vi "ReadTiffPage_text.vi"(0 "TIFF file":T2 {"BigTiff,Endian" items=["Big-Endian"=0, "Native"=1, "Little-Endian"=2, "BigTiff-Big-Endian"=256, "Bigtiff,Native"=257, "Biftiff,Littleendian"=258]}, 2 "IFDoffset":i64, 3 "error in":errorcluster) -> (6 "TIFF file out":T2 {"BigTiff,Endian" items=["Big-Endian"=0, "Native"=1, "Little-Endian"=2, "BigTiff-Big-Endian"=256, "Bigtiff,Native"=257, "Biftiff,Littleendian"=258]}, 8 "string":string, 9 "Next offset":i64, 10 "error out":errorcluster)   [LabVIEW 2011]
uses:
  IFD.ctl
  GetTagValues_U8s.vi
panel:
  out "Byte-Reihenfolge (0:Big-Endian, Netzwerkreihenfolge)":T1(ring)=enum."native, host order"
  out "Directory Entries":T3[](array[typedef])
  out "IFDs":u16
  # "seems to work!"
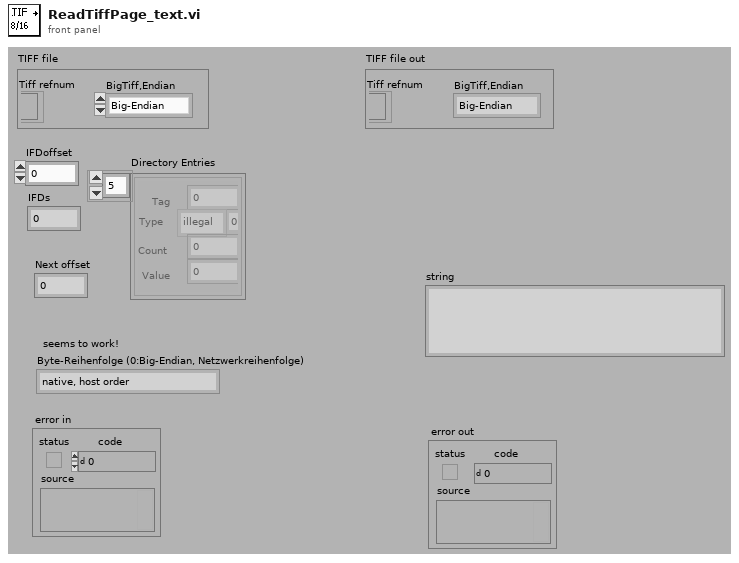
[diagram p1: front panel]
types:
  T1 = enum16{"big-endian, network order", "native, host order", "little-endian"}
  T2 = cluster{"Tiff refnum":refnum<file>, "BigTiff,Endian":u16}
  T3 = typedef "IFD.ctl" = cluster{"Tag":u16, "Type":enum16{"illegal", "Byte", "Ascii", "Short", "Long", "Rational", "SByte", "Undefined", "SShort", "SLong", "SRational 2xSLong", "Float 4byte", "Double 8Byte", "No13", "No14", "No15", "U64", "I64", "U64-IFD8"}, "Count":u64, "Value":u64}
  T4 = cluster{"Tag":u16, "Type":enum16{"illegal", "Byte", "Ascii", "Short", "Long", "Rational", "SByte", "Undefined", "SShort", "SLong", "SRational 2xSLong", "Float 4byte", "Double 8Byte"}, "Count":u32, "Value":u32}
  T5 = cluster{"Tag":u16, "Type":enum16{"illegal", "Byte", "Ascii", "Short", "Long", "Rational", "SByte", "Undefined", "SShort", "SLong", "SRational 2xSLong", "Float 4byte", "Double 8Byte"}, "Count":u32, "Value":u32}[]
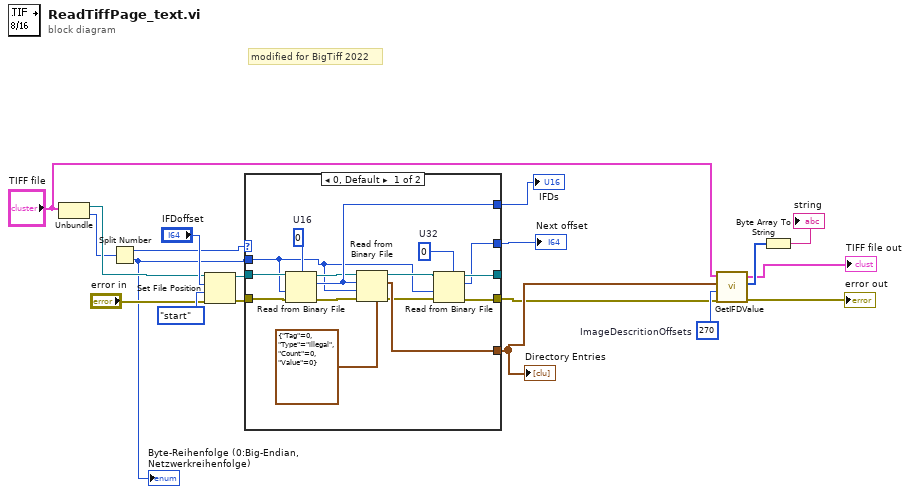
[diagram p0: block diagram]
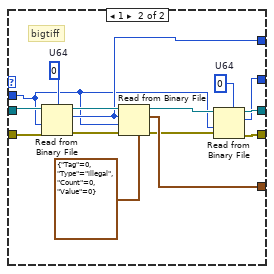
[diagram p2: hidden frame]
diagram:
  w14 = u16 270  # ImageDescritionOffsets
  # "modified for BigTiff 2022"
  n1 = Unbundle("TIFF file") -> ("Tiff refnum"=w16:refnum<file>, "BigTiff,Endian"=w12:u16)
  n2 = Split Number(x=w12) -> (hi(x)=w6:u8, lo(x)=w5:u8)
  "Byte-Reihenfolge (0:Big-Endian, Netzwerkreihenfolge)" <- w5
  n3 = Set File Position(offset (in bytes) (0)="IFDoffset", refnum=w16, from (0:start)=enum16{"start", "end", "current"}."start" ("pos mode (0:2)"), error in="error in") -> (refnum out=w7:refnum<file>, error out=w8:errorcluster)
  n4 = case shown="0, Default" w6 {
    tunnel: [w33 w43] -> w1
    tunnel: w8 -> [w32 w45]
    tunnel: w7 -> [w31 w44]
    tunnel: [w24 w38] -> _
    tunnel: [w23 w40] -> w3
    tunnel: [w28 w42] -> w4
    tunnel: w5 -> [w20 w37]
    tunnel: [w22 w35] -> w2
    frame 0, Default {
      w21 = u32 0  # U32
      w34 = u16 0  # U16
      n5 = Read from Binary File(5:w34, 8:w32, 9:w20, 11:w31) -> (0:w29:errorcluster, 2:w33:u16, 3:w30:refnum<file>)  [unwired: 3 out]
      n6 = Read from Binary File(5:T4 {"Tag"=0, "Type"=enum."illegal", "Count"=0, "Value"=0} ("Cluster"), 8:w29, 9:w20, 10:w33, 11:w30) -> (0:w26:errorcluster, 2:w28:T5, 3:w25:refnum<file>)  [unwired: 2 out]
      n7 = Read from Binary File(5:w21, 8:w26, 9:w20, 11:w25) -> (0:w23:errorcluster, 2:w22:u32, 3:w24:refnum<file>)  [unwired: 3 out]
    }
    frame 1 {
      w36 = u64 0  # U64
      w49 = u64 0  # U64
      # "bigtiff"
      n8 = Read from Binary File(5:w49, 8:w45, 9:w37, 11:w44) -> (0:w47:errorcluster, 2:w43:u64, 3:w48:refnum<file>)  [unwired: 3 out]
      n9 = Read from Binary File(5:T3 {"Tag"=0, "Type"=enum."illegal", "Count"=0, "Value"=0} ("Cluster"), 8:w47, 9:w37, 10:w43, 11:w48) -> (0:w41:errorcluster, 2:w42:T3[], 3:w39:refnum<file>)  [unwired: 2 out]
      n10 = Read from Binary File(5:w36, 8:w41, 9:w37, 11:w39) -> (0:w40:errorcluster, 2:w35:u64, 3:w38:refnum<file>)  [unwired: 3 out]
    }
  }
  "IFDs" <- w1
  "Directory Entries" <- w4
  "Next offset" <- w2
  n11 = call-poly "GetIFDValue.vi"("error in (no error)"=w3, "Tag Code"=w14, "Directory Entries"=w4, "TIFF file"="TIFF file") -> ("error out"=→"error out":errorcluster, "Byte array"=w13:u8[], "TIFF file out"=→"TIFF file out":T2)  [unwired: 3 out]
  n12 = Byte Array To String(unsigned byte array=w13) -> (string=→"string":string)
